vi "SendStopUserEvent.vi"(3 "VI Refnum in":refnum<vi>, 9 "error in":errorcluster) -> (0 "VI Refnum out":refnum<vi>, 6 "error out":errorcluster)   [LabVIEW 2009]
uses:
  Stop.ctl
  StopUserEvent.ctl
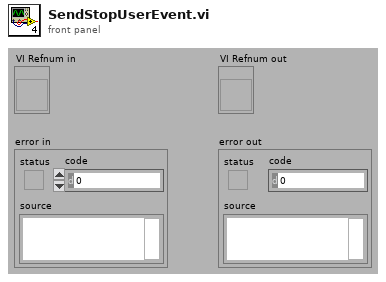
[diagram p1: front panel]
types:
  T1 = typedef "StopUserEvent.ctl" = refnum<user-event>
  T2 = typedef "Stop.ctl" = bool
  T3 = enum32{"Bad", "Idle", "Run top level", "Running"}
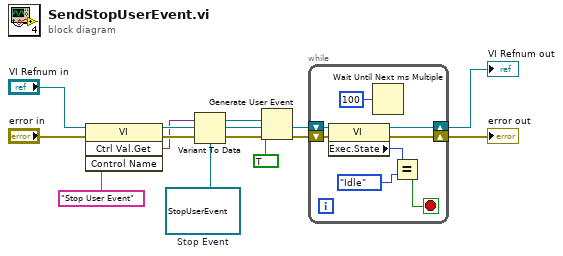
[diagram p0: block diagram]
diagram:
  w13 = T1 refnum  # Stop Event
  n1 = invoke class="VI" method="Ctrl Val.Get"(reference="VI Refnum in", error in="error in", "Control Name"="Stop User Event") -> (reference out=w8:refnum<vi>, error out=w6:errorcluster, "Get Control Value Variant"=w4:variant)  [unwired: 1 in, 1 out]
  n2 = Variant To Data(error in=w6, Variant=w4, type=w13) -> (error out=w7:errorcluster, data=w12:T1)
  n3 = Generate User Event(user event=w12, event data cluster=T2 TRUE ("event data"), error in=w7) -> (error out=w9:errorcluster)  [unwired: 1 out]
  n4 = while {
    shift-right: [w15] -> w11
    shift-left: w8 -> [w21]
    shift-right: [w16] -> w10
    shift-left: w9 -> [w20]
    stop <- w17 stop-if-true
    n5 = property class="VI"(reference=w21, error in=w20) -> (reference out=w15:refnum<vi>, error out=w16:errorcluster, "Exec.State"=w19:T3)
    n6 = Wait Until Next ms Multiple(millisecond multiple=u32 100) -> ()  [unwired: 1 out]
    n7 = Equal?(x=w19, y=T3."Idle" ("Execution:State")) -> (x = y?=w17:bool)
  }
  "VI Refnum out" <- w11
  "error out" <- w10
